vi "Init Actor.vi"() -> (2 "Actor":refnum<class "Actor.lvclass">)   [LabVIEW 2025, in "jettl.lvlib" / "Base Actor.lvlib"]
uses:
  Base Actor.lvlib
  Actor/Actor.lvclass
  Base Actor/Base Actor.lvclass
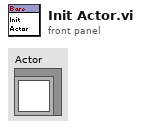
[diagram p1: front panel]
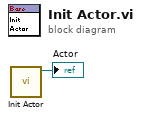
[diagram p0: block diagram]
diagram:
  n1 = call "Init Actor.vi"() -> ("Base Actor out"=→"Actor":refnum<class "Base Actor.lvclass">)  [unwired: 11 in]
